vi "HandleItemActivation.vi"(8 "error in (no error)":errorcluster, 11 "GettingStartedWindow.lvlib:Web.lvclass":refnum<class "Web.lvclass">) -> (0 "error out":errorcluster, 3 "GettingStartedWindow.lvlib:Web.lvclass 2":refnum<class "Web.lvclass">)   [LabVIEW 2009, in "NavScreen.lvlib" / "Web.lvclass"]
uses:
  Web.lvclass
  Web.lvclass/Web.ctl
  <vilib>/Platform/browser.llb/Open URL in Default Browser (string).vi
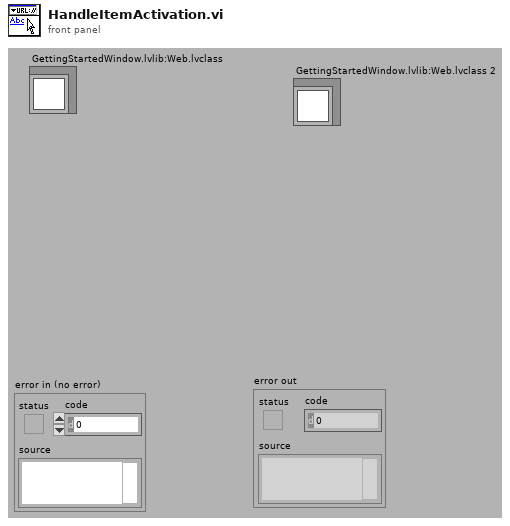
[diagram p1: front panel]
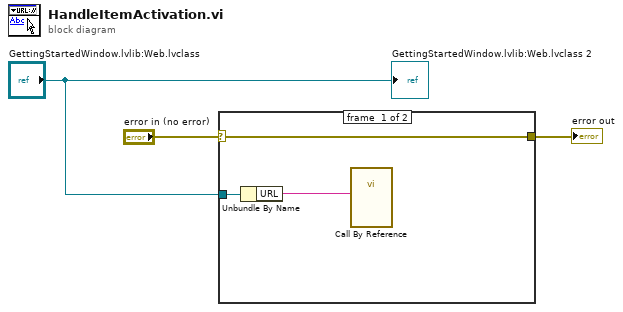
[diagram p0: block diagram]
diagram:
  n1 = case shown="No Error" "error in (no error)" {
    selector: "error in (no error)" -> [w6 w7]
    tunnel: [w6 w7] -> w2
    tunnel: "GettingStartedWindow.lvlib:Web.lvclass" -> [w5 _]
    frame #0 {
      n2 = Unbundle By Name(w5) -> ("URL"=w4:string)
      n3 = call-by-ref "?"("URL"=w4) -> ()  [unwired: 7 in, 4 out]
    }
    frame #1 {
    }
  }
  "error out" <- w2
  "GettingStartedWindow.lvlib:Web.lvclass 2" <- "GettingStartedWindow.lvlib:Web.lvclass"
